vi "PointDir2Lines.vi"(10 "Point":cluster{"X":dbl, "Y":dbl, "Z":dbl}, 11 "DirVecs":dbl[][](array[numeric])) -> (3 "Lines":T1(array[cluster]))   [LabVIEW 2014]
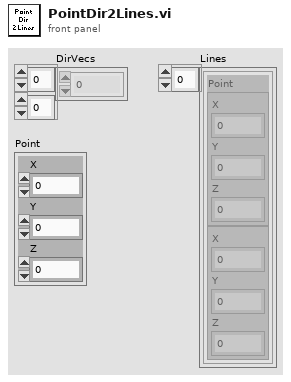
[diagram p1: front panel]
types:
  T1 = cluster{"Point":cluster{"X":dbl, "Y":dbl, "Z":dbl}, cluster{"X":dbl, "Y":dbl, "Z":dbl}}[]
  T2 = cluster{"Point":cluster{"X":dbl, "Y":dbl, "Z":dbl}, cluster{"X":dbl, "Y":dbl, "Z":dbl}}
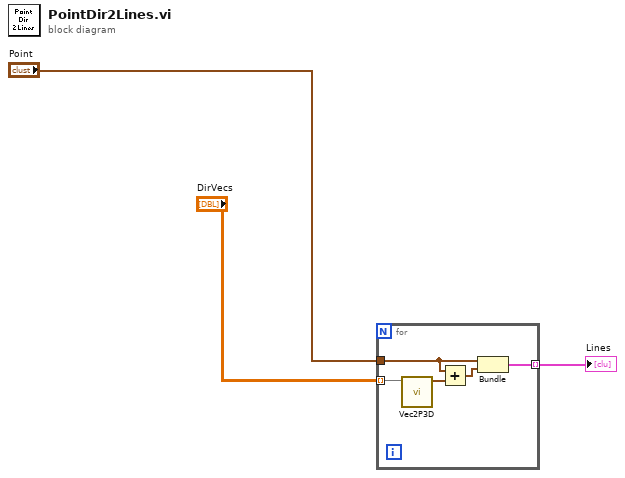
[diagram p0: block diagram]
diagram:
  n1 = for {
    tunnel: "Point" -> [w6]
    tunnel: "DirVecs" -> [w8] mode=indexing
    tunnel: [w4] -> w1 mode=indexing
    n2 = call "Vec2P3D.vi"("Vec"=w8) -> ("P0"=w7:cluster{"X":dbl, "Y":dbl, "Z":dbl})  [unwired: 10 in]
    n3 = Add(x=w6, y=w7) -> (x+y=w5:cluster{"X":dbl, "Y":dbl, "Z":dbl})
    n4 = Bundle("Point"=w6, w5) -> (w4:T2)  [unwired: 1 in]
  }
  "Lines" <- w1
